vi "Ogrod_Warzywny.vi"() -> ()   [LabVIEW 2023]
uses:
  Ogrod_zmienne.vi
panel:
  in  "Ustaw":bool
  in  "Ilosc zraszaczy":dbl
  in  "Rok":dbl
  in  "Miesiac":dbl
  in  "Dzien":dbl
  in  "Minuta":dbl=3.0
  in  "Godzina":dbl=1.0
  in  "Sekcja tryb reczny":dbl
  in  "Czas podlewania":dbl
  in  "Liczba sekcji":dbl=1.0
  in  "Podlewaj tryb reczny":bool
  in  "Podlewaj":bool
  # "Harmonogram"
  # "Automatyczny"
  # "Reczny"
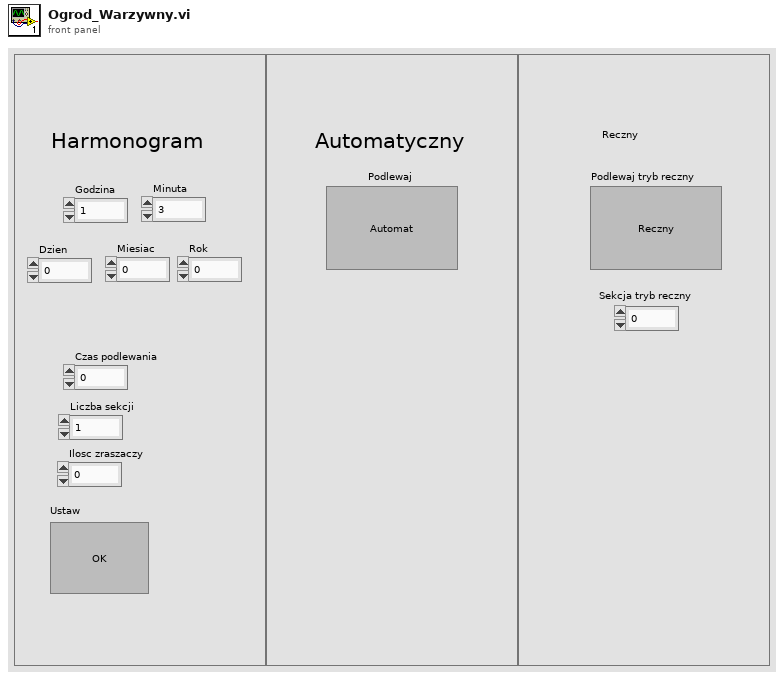
[diagram p1: front panel]
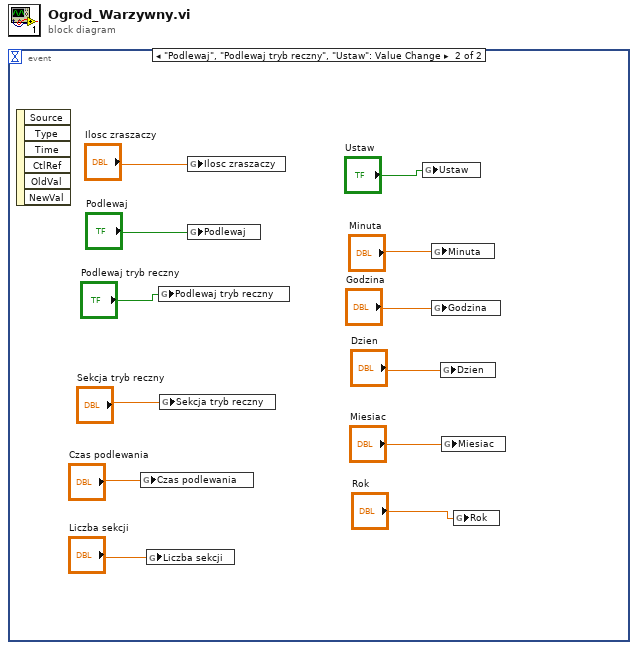
[diagram p0: block diagram]
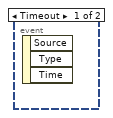
[diagram p2: hidden frame]
diagram:
  n1 = event shown="[1] \"Podlewaj\", \"Podlewaj tryb reczny\", \"Ustaw\": Value Change" {
    selector: _ -> [_ _]
    dyn-events: _ -> [_ _]
    timeout: _ -> [_ _]
    event Timeout {
      n2 = event-data() -> ()  [unwired: 1 in, 3 out]
    }
    event "Podlewaj", "Podlewaj tryb reczny", "Ustaw": Value Change {
      n3 = event-data() -> ()  [unwired: 1 in, 6 out]
      n4 = global write "Ogrod_zmienne.vi" "Czas podlewania"("Czas podlewania") -> ()
      n5 = global write "Ogrod_zmienne.vi" "Liczba sekcji"("Liczba sekcji") -> ()
      n6 = global write "Ogrod_zmienne.vi" "Podlewaj tryb reczny"("Podlewaj tryb reczny") -> ()
      n7 = global write "Ogrod_zmienne.vi" "Sekcja tryb reczny"("Sekcja tryb reczny") -> ()
      n8 = global write "Ogrod_zmienne.vi" "Ilosc zraszaczy"("Ilosc zraszaczy") -> ()
      n9 = global write "Ogrod_zmienne.vi" "Podlewaj"("Podlewaj") -> ()
      n10 = global write "Ogrod_zmienne.vi" "Ustaw"("Ustaw") -> ()
      n11 = global write "Ogrod_zmienne.vi" "Minuta"("Minuta") -> ()
      n12 = global write "Ogrod_zmienne.vi" "Godzina"("Godzina") -> ()
      n13 = global write "Ogrod_zmienne.vi" "Dzien"("Dzien") -> ()
      n14 = global write "Ogrod_zmienne.vi" "Miesiac"("Miesiac") -> ()
      n15 = global write "Ogrod_zmienne.vi" "Rok"("Rok") -> ()
    }
  }
